vi "Chrg_Dschrg_2.vi"(1 "Error log filepath":path, 3 "Strain Offset":dbl, 4 "PS VISA in":refnum<visa-resource-name>, 5 "PS error in":errorcluster caption="PS error in (no error)", 6 "CyclePath":path=path "C:/Users/ga11/Desktop/VI/results/3PtestCharge.lvm" caption="Filename", 7 "Battery Type":T1(ring), 8 "Charge/discharge":enum8{"Charge", "Discharge"}(ring), 9 "Charge/Discharge Voltage Setpoint":dbl format="%#.6g", 11 "Current Setpoint":dbl format="%#.6g", 13 "Current Cutoff":dbl) -> (14 "PS VISA out":refnum<visa-resource-name>, 19 "PS error out":errorcluster)   [LabVIEW 2020]
uses:
  <vilib>/Utility/TradDaqScaling.llb/Convert Strain Gauge Reading (scaler).vi
  Drivers-IT-M3400/IT-M3400.lvlib
panel:
  out "Read Current(A)":dbl format="%.2g"
  out "Read Voltage(V)":dbl format="%.2g"
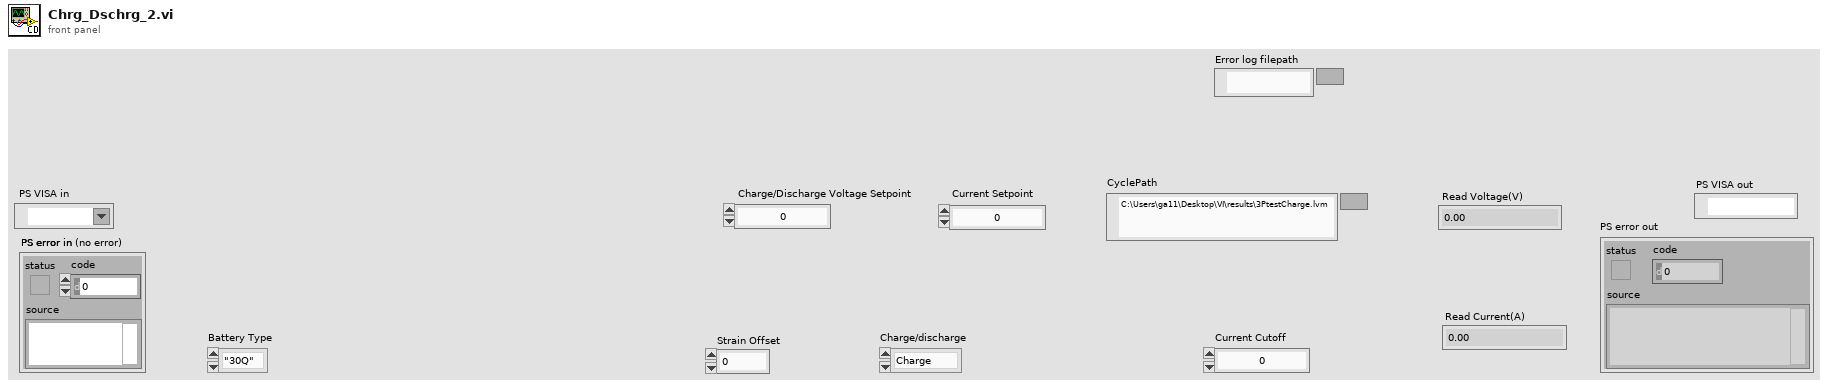
[diagram p1: front panel]
types:
  T1 = enum16{"\"30Q\"", "\"40T\"", "\"2P30Q\"", "\"3P30Q\"", "\"Nissan Leaf\""}
  T2 = cluster{"Baud Rate":u32, "Parity":u16, "Data Bits":u16, "Stop Bits":u16, "Flow Control":u16}
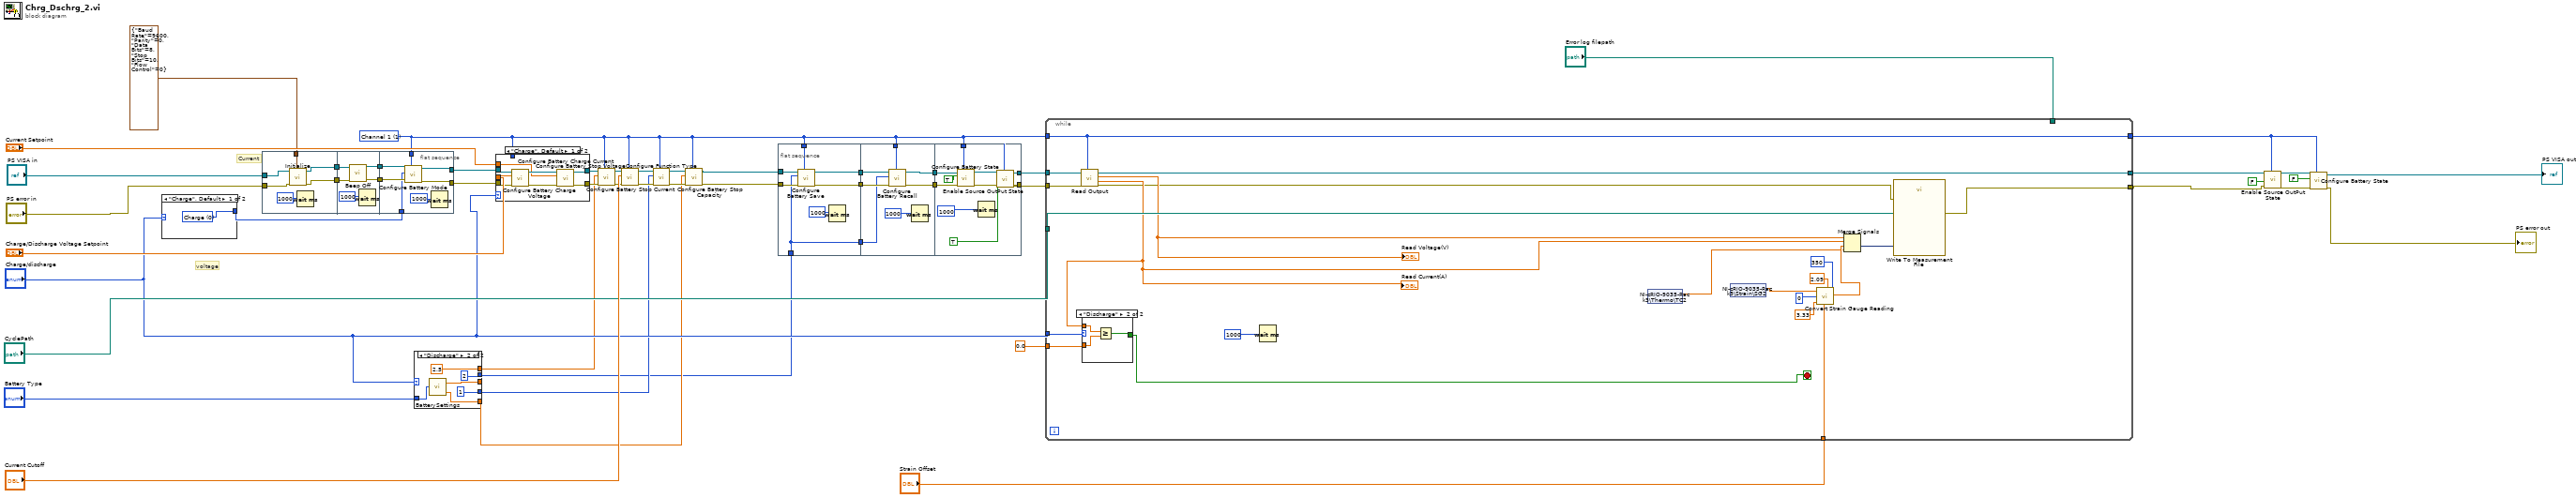
[diagram p0: block diagram]
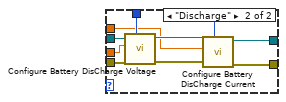
[diagram p2: hidden frame]
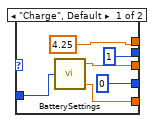
[diagram p3: hidden frame]
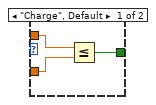
[diagram p4: hidden frame]
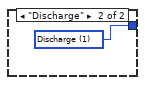
[diagram p5: hidden frame]
diagram:
  w12 = 1 items=["Channel 1"=1, "Channel 2"=2, "Channel 3"=3, "Channel 4"=4, "Channel 5"=5, "Channel 6"=6, "Channel 7"=7, "Channel 8"=8, "Channel 8"=9, "Channel 10"=10, "Channel 11"=11, "Channel 12"=12, "Channel 13"=13, "Channel 14"=14, "Channel 15"=15, "Channel 16"=16] ("Channel")
  # "voltage"
  # "Current"
  n1 = case shown="\"Charge\", Default" "Charge/discharge" {
    tunnel: [w51 w52] -> w20
    frame "Charge", Default {
      w51 = u8 0 items=["Charge", "Discharge"] ("Battery Mode")
    }
    frame "Discharge" {
      w52 = u8 1 items=["Charge", "Discharge"] ("Battery Mode")
    }
  }
  n2 = flat-sequence {
    tunnel: [w54] -> w6
    tunnel: T2 {"Baud Rate"=9600, "Parity"=0, "Data Bits"=8, "Stop Bits"=10, "Flow Control"=0} ("Serial Configuration") -> [w58]
    tunnel: "PS error in" -> [w57]
    tunnel: "PS VISA in" -> [w56]
    tunnel: [w53] -> w5
    tunnel: [w63] -> w35
    tunnel: [w62] -> w34
    tunnel: w6 -> [w61]
    tunnel: w5 -> [w60]
    tunnel: w35 -> [w67]
    tunnel: w34 -> [w69]
    tunnel: w12 -> [w70]
    tunnel: w20 -> [w68]
    tunnel: [w64] -> w9
    tunnel: [w65] -> w8
    frame #0 {
      n3 = call "Initialize.vi"("Serial Configuration"=w58, "error in"=w57, "VISA resource name"=w56) -> ("error out"=w53:errorcluster, "VISA resource name out"=w54:refnum<visa-resource-name>)  [unwired: 7 in]
      n4 = Wait (ms)(milliseconds to wait=1000) -> ()  [unwired: 1 out]
    }
    frame #1 {
      n5 = call "Beep Off.vi"("error in"=w60, "VISA resource name"=w61) -> ("error out"=w62:errorcluster, "VISA resource name out"=w63:refnum<visa-resource-name>)  [unwired: 8 in]
      n6 = Wait (ms)(milliseconds to wait=1000) -> ()  [unwired: 1 out]
    }
    frame #2 {
      n7 = call "Configure Battery Mode.vi"("Channel"=w70, "error in"=w69, "Battery Mode"=w68, "VISA resource name"=w67) -> ("error out"=w64:errorcluster, "VISA resource name out"=w65:refnum<visa-resource-name>)  [unwired: 6 in]
      n8 = Wait (ms)(milliseconds to wait=1000) -> ()  [unwired: 1 out]
    }
  }
  n9 = case shown="\"Discharge\"" "Charge/discharge" {
    tunnel: "Battery Type" -> [w76 w82]
    tunnel: [w75 w80] -> _
    tunnel: [u8 0 ("File") u8 1 ("File")] -> w14
    tunnel: [u8 1 ("File") u8 2 ("File")] -> w11
    tunnel: [w72 w78] -> w13
    tunnel: [4.25 2.5] -> w10
    frame "Charge", Default {
      n10 = call "BatterySettings.vi"("Battery Type"=w76) -> ("RatedCapacity (Ah)"=w72:dbl, "Max Voltage (V)"=w75:dbl)  [unwired: 2 in, 1 out]
    }
    frame "Discharge" {
      n11 = call "BatterySettings.vi"("Battery Type"=w82) -> ("RatedCapacity (Ah)"=w78:dbl, "Min Voltage (V)"=w80:dbl)  [unwired: 2 in, 1 out]
    }
  }
  n12 = case shown="\"Charge\", Default" "Charge/discharge" {
    tunnel: w8 -> [w90 w99]
    tunnel: w9 -> [w89 w98]
    tunnel: [w84 w95] -> w27
    tunnel: [w83 w94] -> w26
    tunnel: w12 -> [_ w93]
    tunnel: "Charge/Discharge Voltage Setpoint" -> [w86 w92]
    tunnel: "Current Setpoint" -> [w85 w91]
    frame "Charge", Default {
      n13 = call "Configure Battery Charge Voltage.vi"("error in"=w89, "Charge Voltage(V)"=w86, "VISA resource name"=w90) -> ("error out"=w87:errorcluster, "VISA resource name out"=w88:refnum<visa-resource-name>)  [unwired: 6 in]
      n14 = call "Configure Battery Charge Current.vi"("error in"=w87, "Charge Current(A)"=w85, "VISA resource name"=w88) -> ("error out"=w83:errorcluster, "VISA resource name out"=w84:refnum<visa-resource-name>)  [unwired: 7 in]
    }
    frame "Discharge" {
      n15 = call "Configure Battery DisCharge Voltage.vi"("Channel"=w93, "error in"=w98, "Discharge Voltage(V)"=w92, "VISA resource name"=w99) -> ("error out"=w96:errorcluster, "VISA resource name out"=w97:refnum<visa-resource-name>)  [unwired: 6 in]
      n16 = call "Configure Battery DisCharge Current.vi"("Channel"=w93, "error in"=w96, "Discharge Current(A)"=w91, "VISA resource name"=w97) -> ("error out"=w94:errorcluster, "VISA resource name out"=w95:refnum<visa-resource-name>)  [unwired: 6 in]
    }
  }
  n17 = call "Configure Battery Stop Voltage.vi"("Channel"=w12, "error in"=w26, "Stop Voltage(V)"=w10, "VISA resource name"=w27) -> ("error out"=w32:errorcluster, "VISA resource name out"=w33:refnum<visa-resource-name>)  [unwired: 6 in]
  n18 = call "Configure Battery Stop Current.vi"("Channel"=w12, "error in"=w32, "Stop Current(A)"="Current Cutoff", "VISA resource name"=w33) -> ("error out"=w16:errorcluster, "VISA resource name out"=w18:refnum<visa-resource-name>)  [unwired: 6 in]
  n19 = call "Configure Function Type.vi"("Channel"=w12, "error in"=w16, "Function Type"=w14, "VISA resource name"=w18) -> ("error out"=w15:errorcluster, "VISA resource name out"=w17:refnum<visa-resource-name>)  [unwired: 6 in]
  n20 = call "Configure Battery Stop Capacity.vi"("Channel"=w12, "error in"=w15, "Stop Capacity(Ah)"=w13, "VISA resource name"=w17) -> ("error out"=w3:errorcluster, "VISA resource name out"=w4:refnum<visa-resource-name>)  [unwired: 6 in]
  n21 = flat-sequence {
    tunnel: w11 -> [w105]
    tunnel: w12 -> [w100]
    tunnel: [w103] -> w40
    tunnel: [w105] -> w39
    tunnel: [w102] -> w38
    tunnel: w3 -> [w106]
    tunnel: w4 -> [w104]
    tunnel: [w109] -> w37
    tunnel: [w110] -> w36
    tunnel: w40 -> [w113]
    tunnel: w39 -> [w112]
    tunnel: w38 -> [w111]
    tunnel: w12 -> [w107]
    tunnel: [w117] -> w25
    tunnel: [w116] -> w24
    tunnel: w12 -> [w115]
    tunnel: w37 -> [w123]
    tunnel: w36 -> [w122]
    frame #0 {
      n22 = call "Configure Battery Save.vi"("Channel"=w100, "error in"=w106, "File"=w105, "VISA resource name"=w104) -> ("error out"=w103:errorcluster, "VISA resource name out"=w102:refnum<visa-resource-name>)  [unwired: 6 in]
      n23 = Wait (ms)(milliseconds to wait=1000) -> ()  [unwired: 1 out]
    }
    frame #1 {
      n24 = call "Configure Battery Recall.vi"("Channel"=w107, "error in"=w113, "File"=w112, "VISA resource name"=w111) -> ("error out"=w110:errorcluster, "VISA resource name out"=w109:refnum<visa-resource-name>)  [unwired: 6 in]
      n25 = Wait (ms)(milliseconds to wait=1000) -> ()  [unwired: 1 out]
    }
    frame #2 {
      n26 = call "Configure Battery State.vi"("Channel"=w115, "error in"=w122, "State"=TRUE, "VISA resource name"=w123) -> ("error out"=w120:errorcluster, "VISA resource name out"=w121:refnum<visa-resource-name>)  [unwired: 6 in]
      n27 = Wait (ms)(milliseconds to wait=1000) -> ()  [unwired: 1 out]
      n28 = call "Enable Source OutPut State.vi"("Channel"=w115, "error in"=w120, "State"=TRUE ("Enable Output|Intput"), "VISA resource name"=w121) -> ("error out"=w116:errorcluster, "VISA resource name out"=w117:refnum<visa-resource-name>)  [unwired: 6 in]
    }
  }
  n29 = while {
    tunnel: [w138] -> w23
    tunnel: [w126] -> w1
    tunnel: w25 -> [w145]
    tunnel: w24 -> [w144]
    tunnel: w12 -> [w137]
    tunnel: [w137] -> w22
    tunnel: "CyclePath" -> [w142]
    tunnel: 0.0 -> [w140]
    tunnel: "Charge/discharge" -> [w139]
    tunnel: "Strain Offset" -> [w132]
    tunnel: "Error log filepath" -> [_]
    stop <- w128 stop-if-true
    n30 = call "Read Output.vi"("Channel"=w137, "error in"=w144, "VISA resource name"=w145) -> ("error out"=w127:errorcluster, "Read Current(A)"=w129:dbl, "Read Voltage(V)"=w130:dbl, "VISA resource name out"=w138:refnum<visa-resource-name>)  [unwired: 5 in]
    "Read Voltage(V)" <- w130
    "Read Current(A)" <- w129
    n31 = case shown="\"Discharge\"" w139 {
      tunnel: w140 -> [w147 w150]
      tunnel: w129 -> [w148 w151]
      tunnel: [w146 w149] -> w128
      frame "Charge", Default {
        n32 = Less Or Equal?(x=w148, y=w147) -> (x <= y?=w146:bool)
      }
      frame "Discharge" {
        n33 = Greater Or Equal?(x=w151, y=w150) -> (x >= y?=w149:bool)
      }
    }
    n34 = Wait (ms)(milliseconds to wait=1000) -> ()  [unwired: 1 out]
    n35 = shared-variable "NI-cRIO-9035-Rack3\\Thermo\\TC2"() -> (w124:dbl)  [unwired: 1 in, 1 out]
    n36 = shared-variable "NI-cRIO-9035-Rack3\\Strain\\SG2"() -> (w131:dbl)  [unwired: 1 in, 1 out]
    n37 = call-poly <vilib>:"Convert Strain Gauge Reading.vi"("Vsg (0.0)"=w131, "Bridge Configuration\n(3:Half Bridge II)"=0, "Vex (3.33)"=3.33, "Vinit (0.0)"=w132, "GF (2.0)"=2.09, "Rg (120)"=350) -> ("Strain"=w125:sgl)  [unwired: 4 in]
    n38 = Merge Signals "Merge Signals"(w130, w129, w125, w124) -> (w143:dynamicdata)
    n39 = call "Write To Measurement File"("Signals"=w143, "error in (no error)"=w127, "Filename"=w142) -> ("error out"=w126:errorcluster)  [unwired: 14 in, 2 out]
  }
  n40 = call "Enable Source OutPut State.vi"("Channel"=w22, "error in"=w1, "State"=FALSE, "VISA resource name"=w23) -> ("error out"=w30:errorcluster, "VISA resource name out"=w31:refnum<visa-resource-name>)  [unwired: 6 in]
  n41 = call "Configure Battery State.vi"("Channel"=w22, "error in"=w30, "State"=FALSE, "VISA resource name"=w31) -> ("error out"=→"PS error out":errorcluster, "VISA resource name out"=→"PS VISA out":refnum<visa-resource-name>)  [unwired: 6 in]
